vi "Debug.vi"(10 "Method":string, 11 "jettl in":refnum<class "jettl.lvclass">) -> (3 "jettl out":refnum<class "jettl.lvclass">)   [LabVIEW 2021, in "jettl.lvlib" / "jettl.lvclass"]
uses:
  jettl.lvclass
panel:
  out "error out":errorcluster
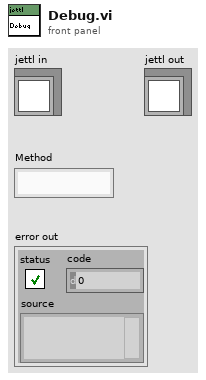
[diagram p1: front panel]
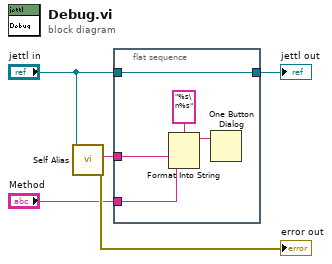
[diagram p0: block diagram]
diagram:
  n1 = call-dynamic "Self Alias.vi"("jettl in"="jettl in") -> ("error out"=→"error out":errorcluster, "Alias"=w3:string)  [unwired: 9 in]
  n2 = flat-sequence {
    tunnel: [w10] -> w5
    tunnel: "jettl in" -> [w10]
    tunnel: "Method" -> [w6]
    tunnel: w3 -> [w7]
    frame #0 {
      n3 = Format Into String(format string="%s\n%s", w7, w6) -> (resulting string=w8:string)  [unwired: 2 in, 1 out]
      n4 = One Button Dialog(message=w8) -> ()  [unwired: 1 in, 1 out]
    }
  }
  "jettl out" <- w5
